vi "Phasor Explorer Lifetime at UC Intersection (discrete).vi"(8 "Error In":errorcluster, 11 "Data for Pseudo UC Intersections":T1={"Linear Coefficients"={"u"=0.0, "v"=0.0}, "Decay Definition"={"offset: t0"=0.0, "period: T"=0.0, "lifetime: tau"=0.0, "Incident Signal: I"=0.0, "Normalized Decays"=FALSE, "IRF Model"=enum."Dirac", "IRF Parameter 1"=0.0, "Poisson Signal"=FALSE}, "Gates Definitions"={"First Gate: t1"=0.0, "Gate Width: W"=0.0, "Gate Step: d"=0.0, "# Gates: G"=0.0, "Use Gate Center"=FALSE, "Frames/Image: F"=0, "Gates/Frame: L"=0, "Bits/Frame: q"=0, "Multiplicity: p"=0, "Gate Type"=enum."Square", "Gate Edge s"=4.0, "Gate Top Slope"=4.0, "Reversed Sawtooth?"=FALSE, "Computation"=FALSE, "User-defined Gate"={"X Array"=[], "Y Array"=[]}, "Tolerance"=50.0, "Integration"=enum."Item 0", "# Steps"=50.0, "Type of User-defined Function"=enum."Gate"}, "iw"=0.0+0.0i, "Phasor Calculation"=enum."Direct Sum"}) -> (0 "Error Out":errorcluster, 1 "Analytical Solution 1":dbl[unit], 3 "Analytical Solution 2":dbl[unit])   [LabVIEW 2021, in "Phasor Explorer.lvlib"]
uses:
  Phasor Explorer.lvlib
  Phasor Gate Definitions.ctl
  Phasor.lvlib
  Phasor Decay Definiton.ctl
  Phasor Calculation Type.ctl
  Phasor Data for SEPL Intersections.ctl
  Phasor Gate Type.ctl
  Phasor IRF Model.ctl
  Graphs/XY Graph/XY Plot Data.ctl
  Graphs/XY Graph/XY Graph Add-Ons.lvlib
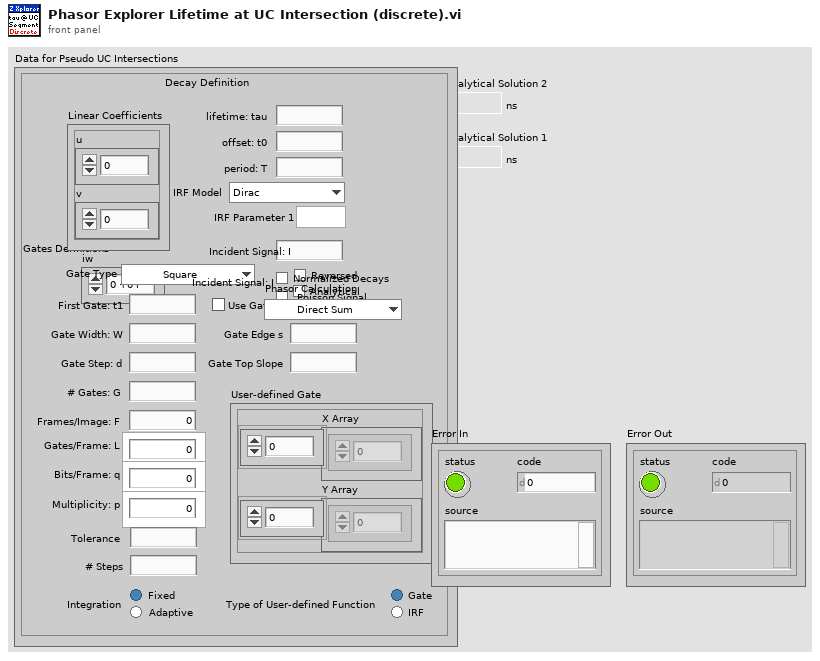
[diagram p1: front panel]
types:
  T1 = typedef "Phasor.lvlib/Phasor Data for SEPL Intersections.ctl" = cluster{"Linear Coefficients":cluster{"u":dbl, "v":dbl}, "Decay Definition":T2, "Gates Definitions":T4, "iw":cdb, "Phasor Calculation":T7}
  T2 = typedef "Phasor.lvlib/Phasor Decay Definiton.ctl" = cluster{"offset: t0":ext, "period: T":ext, "lifetime: tau":ext, "Incident Signal: I":ext, "Normalized Decays":bool, "IRF Model":T3, "IRF Parameter 1":ext, "Poisson Signal":bool}
  T3 = typedef "Phasor.lvlib/Phasor IRF Model.ctl" = enum16{"Dirac", "Exponential"}
  T4 = typedef "Phasor.lvlib/Phasor Gate Definitions.ctl" = cluster{"First Gate: t1":ext, "Gate Width: W":ext, "Gate Step: d":ext, "# Gates: G":ext, "Use Gate Center":bool, "Frames/Image: F":i32, "Gates/Frame: L":i32, "Bits/Frame: q":i32, "Multiplicity: p":i32, "Gate Type":T5, "Gate Edge s":ext, "Gate Top Slope":ext, "Reversed Sawtooth?":bool, "Computation":bool, "User-defined Gate":T6, "Tolerance":ext, "Integration":enum32{"Item 0", "Item 1"}, "# Steps":ext, "Type of User-defined Function":enum32{"Gate", "IRF"}}
  T5 = typedef "Phasor.lvlib/Phasor Gate Type.ctl" = enum16{"Square", "Finite Edge Square", "Finite Edge, Tilted Top Square", "Triangle", "Sawtooth", "User-defined"}
  T6 = typedef "XY Graph Add-Ons.lvlib/XY Plot Data.ctl" = cluster{"X Array":dbl[], "Y Array":dbl[]}
  T7 = typedef "Phasor.lvlib/Phasor Calculation Type.ctl" = enum16{"Direct Sum", "Analytical Formula"}
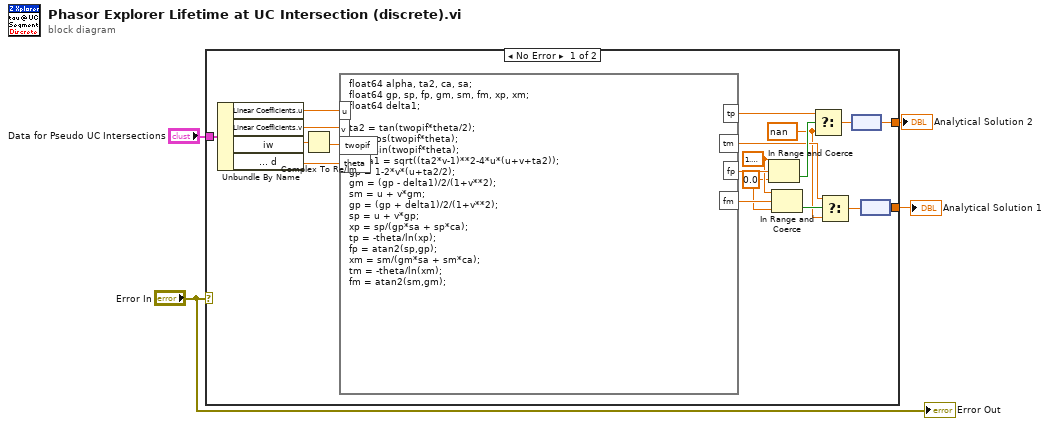
[diagram p0: block diagram]
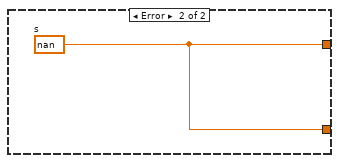
[diagram p2: hidden frame]
diagram:
  n1 = case shown="No Error" "Error In" {
    tunnel: "Data for Pseudo UC Intersections" -> [w23 _]
    tunnel: [w18 w24] -> w3
    tunnel: [w17 w24] -> w2
    frame No Error {
      w5 = nan ("f")
      w9 = 0.0 ("lower limit")
      w10 = 1.5707963267948966
      n2 = Unbundle By Name(w23) -> ("Linear Coefficients.u"=w22:dbl, "Linear Coefficients.v"=w21:dbl, "iw"=w20:cdb, "Gates Definitions.Gate Step: d"=w16:ext)
      n3 = Complex To Re/Im(x + iy=w20) -> (y=w19:dbl)  [unwired: 1 out]
      n4 = formula code="float64 alpha, ta2, ca, sa;\nfloat64 gp, sp, fp, gm, sm, fm, xp, xm;\nfloat64 delta1;\n\nta2 = tan(twopif*theta/2);\nca= cos(twopif*theta);\nsa = sin(twopif*theta);\ndelta1 = sqrt((ta2*v-1)**2-4*u*(u+v+ta2));\ngp = 1-2*v*(u+ta2/2);\ngm = (gp - delta1)/2/(1+v**2);\nsm = u + v*gm;\ngp = (gp + delta1)/2/(1+v**2);\nsp = u + v*gp;\nxp = sp/(gp*sa + sp*ca);\ntp = -theta/ln(xp);\nfp = atan2(sp,gp);\nxm = sm/(gm*sa + sm*ca);\ntm = -theta/ln(xm);\nfm = atan2(sm,gm);"("u"=w22, "v"=w21, "twopif"=w19, "theta"=w16) -> ("tp"=w13:dbl, "tm"=w7:dbl, "fp"=w15:dbl, "fm"=w11:dbl)
      n5 = In Range and Coerce(upper limit=w10, x=w15, lower limit=w9) -> (In Range?=w14:bool)  [unwired: 1 out]
      n6 = In Range and Coerce(upper limit=w10, x=w11, lower limit=w9) -> (In Range?=w8:bool)  [unwired: 1 out]
      n7 = Select(t=w13, s=w14, f=w5) -> (s? t:f=w12:dbl)
      n8 = Select(t=w7, s=w8, f=w5) -> (s? t:f=w6:dbl)
      n9 = node(w12) -> (w17:dbl[unit])
      n10 = node(w6) -> (w18:dbl[unit])
    }
    frame Error {
      w24 = dbl[unit] nan  # s
    }
  }
  "Analytical Solution 1" <- w3
  "Analytical Solution 2" <- w2
  "Error Out" <- "Error In"
